vi "rename channel.vi"(7 "owner ID":string, 8 "error in":errorcluster, 9 "new name":string, 10 "old name":string, 11 "engine configuration in":refnum<class "base TBM sequencer configuration.lvclass">) -> (0 "error out":errorcluster, 3 "engine configuration out":refnum<class "base TBM sequencer configuration.lvclass">)   [LabVIEW 2014, in "base TBM sequencer configuration.lvclass"]
uses:
  base TBM sequencer configuration.lvclass
  <vilib>/NI/Tag Bus/tag/tag descriptor.lvclass
  <vilib>/NI/Tag Bus Module Framework/channel/TBM channel.lvclass
  <vilib>/NI/Configuration Framework/NISE_CEF_TreeControl.lvlib
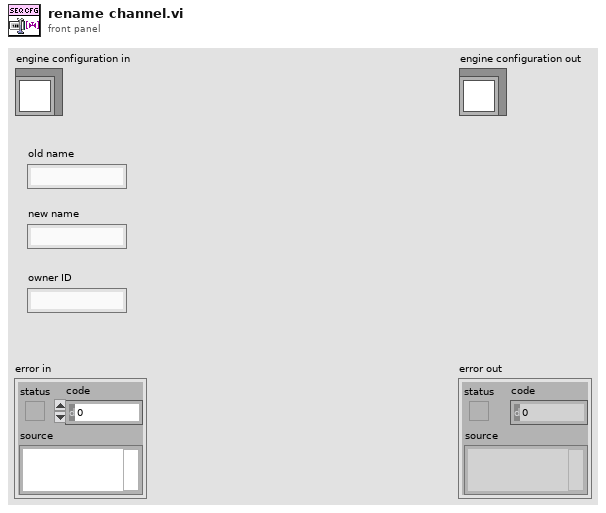
[diagram p1: front panel]
types:
  T1 = typedef "base TBM sequencer configuration.lvclass/Tag Info.ctl" = cluster{"Channel":refnum<class "TBM channel.lvclass">, "Writers":string[], "Readers":string[], "Owning ID":string}
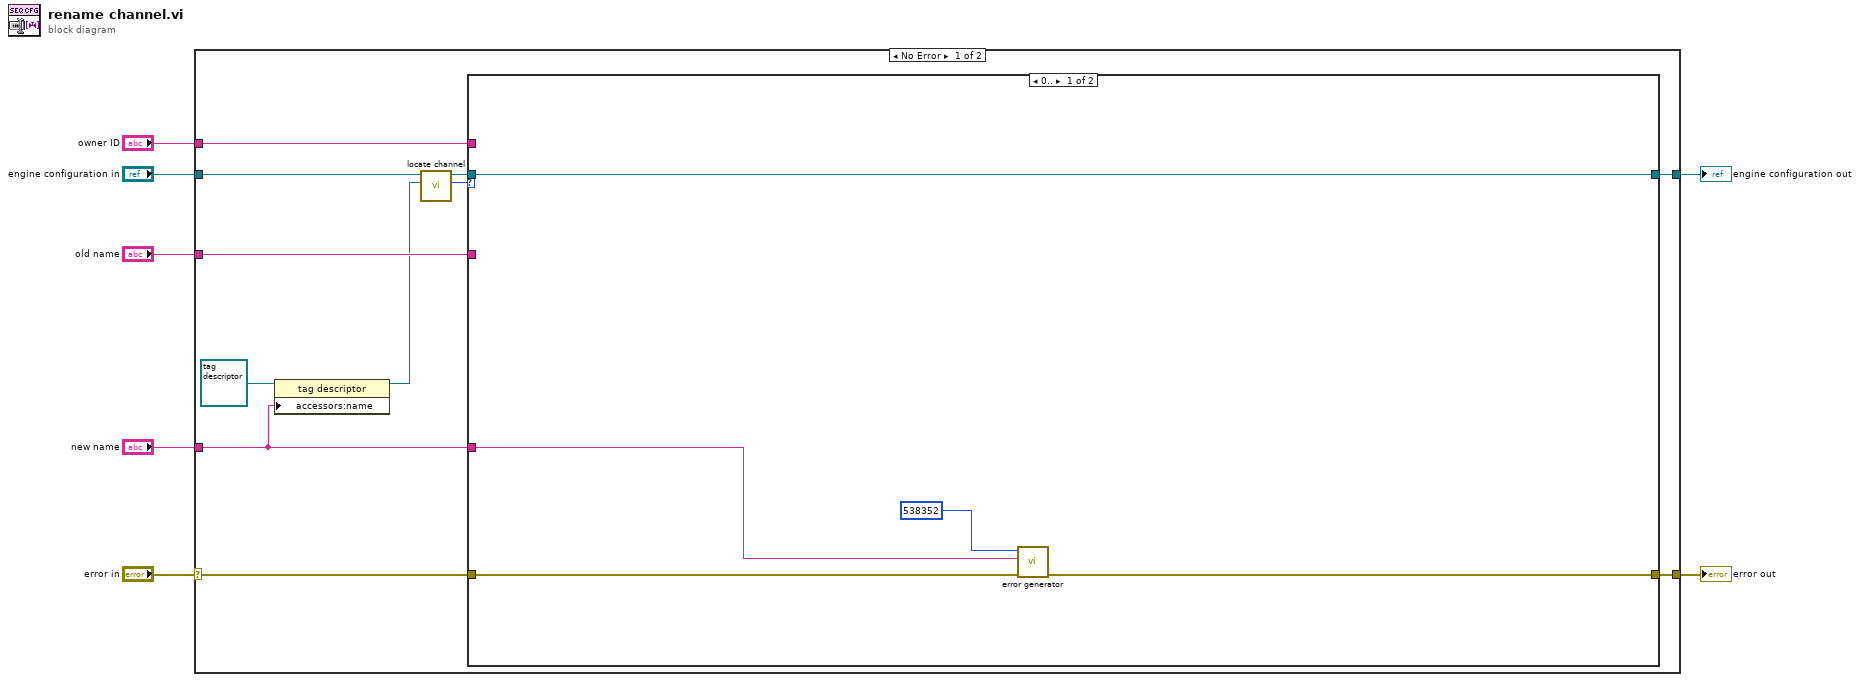
[diagram p0: block diagram]
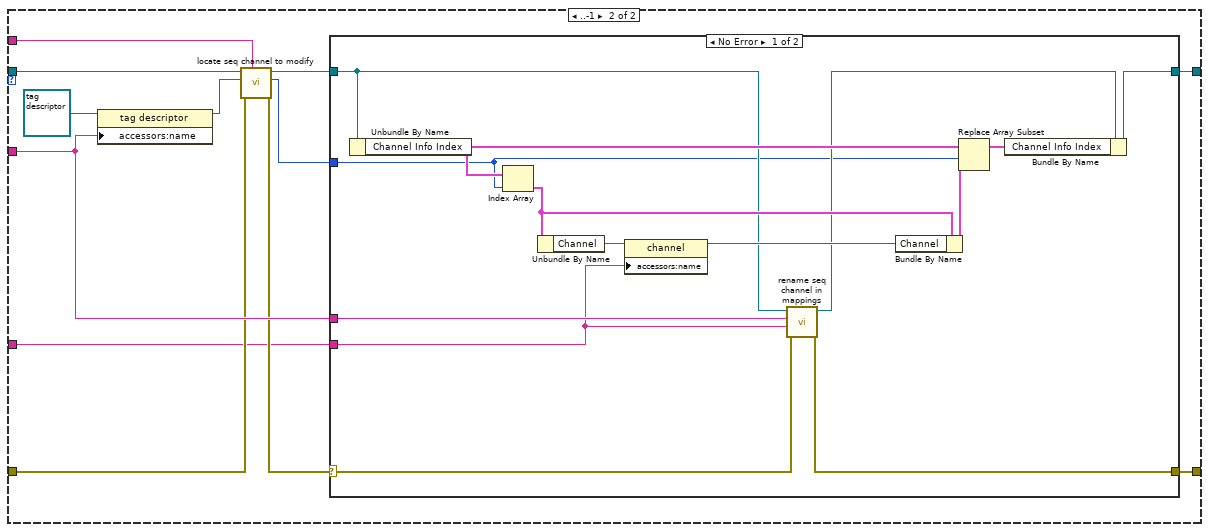
[diagram p2: hidden frame]
diagram:
  n1 = case shown="No Error" "error in" {
    selector: "error in" -> [w14 w53]
    tunnel: [w18 w53] -> w6
    tunnel: [w17 w52] -> w4
    tunnel: "engine configuration in" -> [w13 w52]
    tunnel: "old name" -> [w16 _]
    tunnel: "new name" -> [w10 _]
    tunnel: "owner ID" -> [w15 _]
    frame No Error {
      n2 = property class="tag descriptor"(reference=refnum<class "tag descriptor.lvclass"> refnum ("tag descriptor"), "accessors:name"=w10) -> (reference out=w9:refnum<class "tag descriptor.lvclass">)  [unwired: 1 in, 1 out]
      n3 = call "locate channel.vi"("tag descriptor"=w9, "sequencer config in"=w13) -> ("index"=w8:i32, "sequencer config out"=w12:refnum<class "base TBM sequencer configuration.lvclass">)  [unwired: 8 in]
      n4 = case shown="0.." w8 {
        tunnel: [w21 w34] -> w18
        tunnel: [w23 w33] -> w17
        tunnel: w16 -> [_ w32]
        tunnel: w15 -> [_ w30]
        tunnel: w14 -> [w22 w28]
        tunnel: w12 -> [w23 w25]
        tunnel: w10 -> [w20 w24]
        frame 0.. {
          n5 = call <vilib>:"error generator.vi"("error in"=w22, "append error message"=w20, "error code (0)"=538352) -> ("error out"=w21:errorcluster)  [unwired: 6 in]
        }
        frame ..-1 {
          n6 = property class="tag descriptor"(reference=refnum<class "tag descriptor.lvclass"> refnum ("tag descriptor"), "accessors:name"=w32) -> (reference out=w29:refnum<class "tag descriptor.lvclass">)  [unwired: 1 in, 1 out]
          n7 = call "locate seq channel to modify.vi"("owner ID"=w30, "error in"=w28, "tag descriptor"=w29, "engine configuration in"=w25) -> ("error out"=w27:errorcluster, "index"=w26:i32, "engine configuration out"=w31:refnum<class "base TBM sequencer configuration.lvclass">)  [unwired: 5 in]
          n8 = case shown="No Error" w27 {
            selector: w27 -> [w37 w50]
            tunnel: [w40 w50] -> w34
            tunnel: w31 -> [w42 w51]
            tunnel: [w43 w51] -> w33
            tunnel: w24 -> [w38 _]
            tunnel: w32 -> [w39 _]
            tunnel: w26 -> [w36 _]
            frame No Error {
              n9 = Unbundle By Name(w42) -> ("Channel Info Index"=w45:T1[])
              n10 = Index Array(array=w45, index=w36) -> (element=w48:T1)
              n11 = Unbundle By Name(w48) -> ("Channel"=w49:refnum<class "TBM channel.lvclass">)
              n12 = property class="channel"(reference=w49, "accessors:name"=w38) -> (reference out=w47:refnum<class "TBM channel.lvclass">)  [unwired: 1 in, 1 out]
              n13 = call "rename seq channel in mappings.vi"("error in"=w37, "new seq channel name"=w38, "old seq channel name"=w39, "engine configuration in"=w42) -> ("error out"=w40:errorcluster, "engine configuration out"=w41:refnum<class "base TBM sequencer configuration.lvclass">)  [unwired: 6 in]
              n14 = Bundle By Name(cluster=w48, "Channel"=w47) -> (w46:T1)
              n15 = Replace Array Subset(array=w45, new element=w46, index=w36) -> (w44:T1[])
              n16 = Bundle By Name(cluster=w41, "Channel Info Index"=w44) -> (w43:refnum<class "base TBM sequencer configuration.lvclass">)
            }
            frame Error {
            }
          }
        }
      }
    }
    frame Error {
    }
  }
  "error out" <- w6
  "engine configuration out" <- w4
